vi "Move Key.vi"(4 "Overwrite excisting? [F]":bool, 5 "Key name":string, 6 "New section name":string, 7 "Section name":string, 8 "error in (no error)":errorcluster, 9 "Use Key Regex? [F]":bool, 10 "Use Section Regex? [F]":bool, 11 "Carya Config in":refnum<class "Carya Config.lvclass">) -> (0 "error out":errorcluster, 1 "Moved items":i32, 3 "Carya Config out":refnum<class "Carya Config.lvclass">)   [LabVIEW 2013, in "Carya Config.lvclass"]
doc: "Copyright 2018, Carya Automatisering, Wiebe Walstra."
uses:
  Carya Config.lvclass
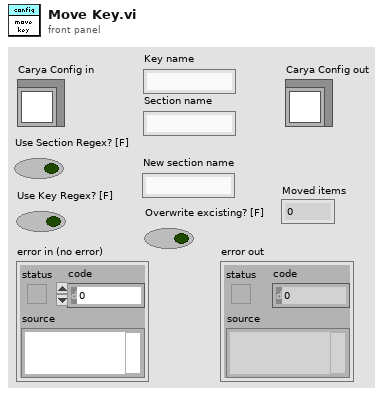
[diagram p1: front panel]
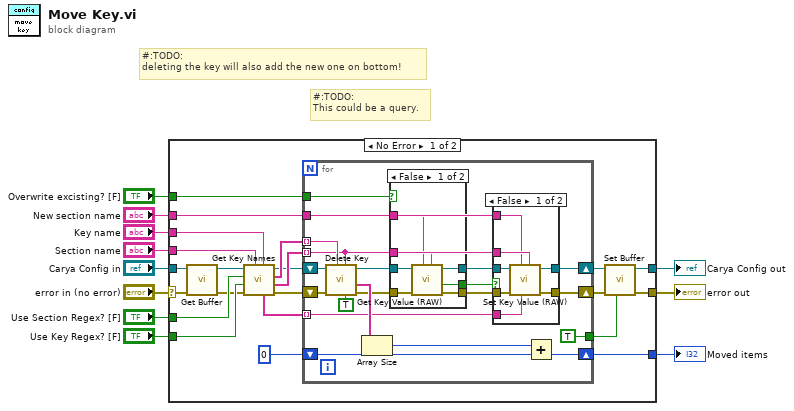
[diagram p0: block diagram]
diagram:
  # "#:TODO:\nThis could be a query."
  # "#:TODO:\ndeleting the key will also add the new one on bottom!"
  n1 = case shown="No Error" "error in (no error)" {
    selector: "error in (no error)" -> [w33 w73]
    tunnel: [w19 w73] -> w10
    tunnel: [w18 w72] -> w8
    tunnel: "Carya Config in" -> [w16 w72]
    tunnel: "Section name" -> [w32 _]
    tunnel: "Key name" -> [w30 _]
    tunnel: [w23 _] -> w5
    tunnel: "Use Section Regex? [F]" -> [w31 _]
    tunnel: "Use Key Regex? [F]" -> [w29 _]
    tunnel: "New section name" -> [w21 _]
    tunnel: "Overwrite excisting? [F]" -> [w20 _]
    frame No Error {
      n2 = call-dynamic "Get Buffer.vi"("error in (no error)"=w33, "Carya Config in"=w16) -> ("error out"=w17:errorcluster, "Config"=w14:refnum<class "Carya Config.lvclass">)  [unwired: 8 in]
      n3 = call-dynamic "Get Key Names.vi"("Key name/Regex"=w30, "Section name/Regex"=w32, "error in (no error)"=w17, "Use Key Regex? [F]"=w29, "Use Section Regex? [F]"=w31, "Carya Config in"=w14) -> ("error out"=w25:errorcluster, "Key names"=w27:string[], "Section names"=w28:string[], "Carya Config out"=w26:refnum<class "Carya Config.lvclass">, "Context (concatenated)"=w13:string[])  [unwired: 1 in]
      n4 = for {
        tunnel: w28 -> [w41] mode=indexing
        tunnel: w27 -> [w38] mode=indexing
        shift-right: [w50] -> w15
        shift-left: w26 -> [w53]
        shift-right: [w51] -> w24
        shift-left: w25 -> [w52]
        shift-right: [w48] -> w23
        shift-left: 0 -> [w47]
        tunnel: w21 -> [w42]
        tunnel: w20 -> [w40]
        tunnel: w13 -> [w37] mode=indexing
        tunnel: [TRUE] -> w12
        n5 = call-dynamic "Delete Key.vi"("Return deleted names? [F]"=TRUE, "Key name"=w38, "Section name"=w41, "error in (no error)"=w52, "Carya Config in"=w53) -> ("error out"=w45:errorcluster, "Key names"=w49:string[], "Carya Config out"=w46:refnum<class "Carya Config.lvclass">)  [unwired: 3 in, 1 out]
        n6 = Array Size(array=w49) -> (size(s)=w36:i32)
        n7 = case shown="False" w40 {
          tunnel: w46 -> [w69 w71]
          tunnel: w45 -> [w68 w70]
          tunnel: [w64 w71] -> w44
          tunnel: [w65 w70] -> w43
          tunnel: w42 -> [w67 _]
          tunnel: w38 -> [w66 _]
          tunnel: [w63 _] -> w39
          frame False {
            n8 = call-dynamic "Get Key Value (RAW).vi"("Key name"=w66, "Section name"=w67, "error in (no error)"=w68, "Carya Config in"=w69) -> ("error out"=w65:errorcluster, "Found?"=w63:bool, "Carya Config out"=w64:refnum<class "Carya Config.lvclass">)  [unwired: 4 in, 1 out]
          }
          frame True {
          }
        }
        n9 = case shown="False" w39 {
          tunnel: [w60 w61] -> w51
          tunnel: [w59 w62] -> w50
          tunnel: w44 -> [w58 w62]
          tunnel: w43 -> [w57 w61]
          tunnel: w42 -> [w54 _]
          tunnel: w38 -> [w55 _]
          tunnel: w37 -> [w56 _]
          frame False {
            n10 = call-dynamic "Set Key Value (RAW).vi"("Key name"=w55, "Key value"=w56, "Section name"=w54, "error in (no error)"=w57, "Carya Config in"=w58) -> ("error out"=w60:errorcluster, "Carya Config out"=w59:refnum<class "Carya Config.lvclass">)  [unwired: 2 in, 3 out]
          }
          frame True {
          }
        }
        n11 = Add(x=w36, y=w47) -> (x+y=w48:i32)
      }
      n12 = call-dynamic "Set Buffer.vi"("Set? [T]"=w12, "error in (no error)"=w24, "Carya Config"=w15) -> ("error out"=w19:errorcluster, "Carya Config out"=w18:refnum<class "Carya Config.lvclass">)  [unwired: 7 in]
    }
    frame Error {
    }
  }
  "error out" <- w10
  "Carya Config out" <- w8
  "Moved items" <- w5
